vi "pace measurement_mso7014b.vi"(8 "error in (no error)":errorcluster, 11 "VISA resource name":refnum<visa-resource-name>) -> (0 "CH3 Waveform":waveform(dbl)(graph), 1 "CH1 Waveform":waveform(dbl)(graph), 2 "添加的数组":waveform(dbl)[](array[waveform]))   [LabVIEW 2016]
uses:
  <instrlib>/Agilent 6000 Series/Public/Data/Read Waveform Measurement.vi
  <instrlib>/Agilent 6000 Series/Agilent 6000 Series.lvlib
panel:
  out "Pluse Frequency":dbl
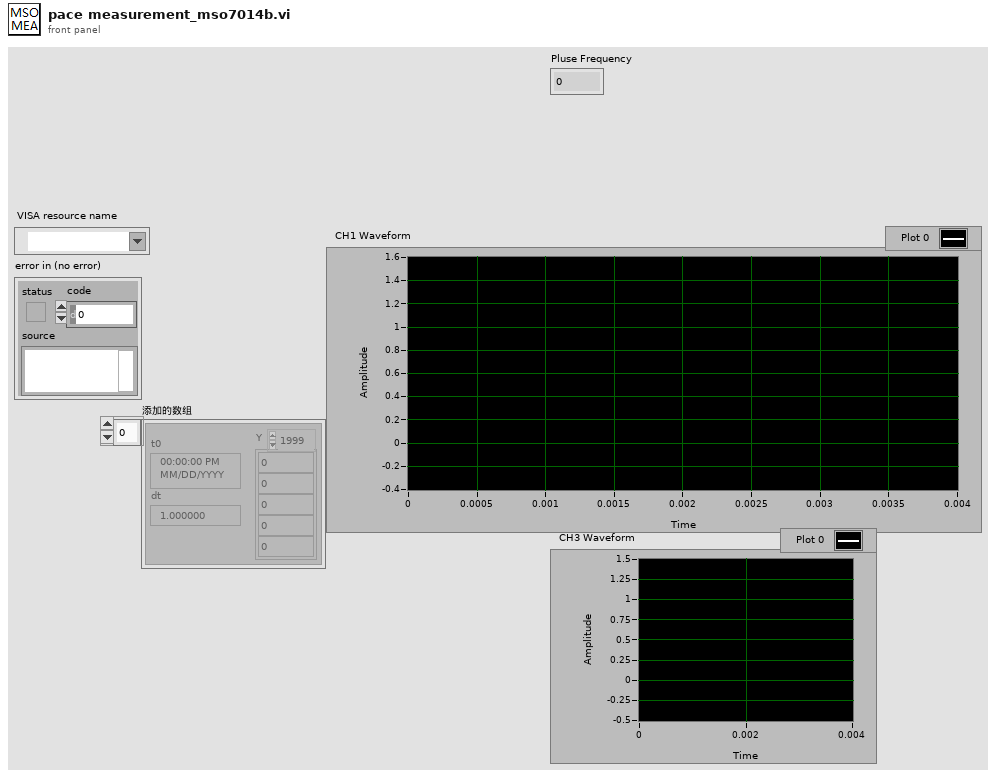
[diagram p1: front panel]
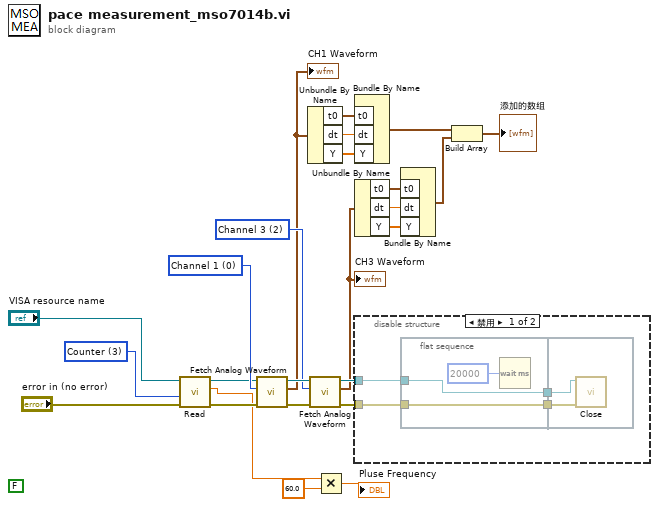
[diagram p0: block diagram]
diagram:
  w8 = u16 3 items=["Amplitude", "Voltage Average", "Base", "Counter", "Delay", "Duty Cycle", "Fall Time", "Frequency", "Voltage Max", "Voltage Min", "Overshoot", "Voltage Vpp", "Period", "Phase", "Preshoot", "Rise Time", "Voltage RMS", "Top", "Width Positive", "X at Max Y", "X at Min Y"] ("Measurement Function (7: Frequency)")
  (unwired) FALSE ("Continuous Acquisition Mode (T: Enable)")
  w23 = u16 2 items=["Channel 1", "Channel 2", "Channel 3", "Channel 4", "Math"] ("Source (0: Channel 1)")
  w25 = u16 0 items=["Channel 1", "Channel 2", "Channel 3", "Channel 4", "Math"] ("Source (0: Channel 1)")
  n1 = call-poly <instrlib>:"Read.vi"("error in (no error)"="error in (no error)", "Measurement Function (7: Frequency)"=w8, "VISA resource name"="VISA resource name") -> ("error out"=w4:errorcluster, "Measured Value"=w3:dbl, "VISA resource name out"=w6:refnum<visa-resource-name>)  [unwired: 6 in]
  n2 = call <instrlib>:"Fetch Analog Waveform.vi"("error in (no error)"=w4, "Source (0: Channel 1)"=w25, "VISA resource name"=w6) -> ("error out"=w20:errorcluster, "Waveform Data"=w19:waveform(dbl), "VISA resource name out"=w24:refnum<visa-resource-name>)  [unwired: 6 in]
  "CH1 Waveform" <- w19
  n3 = Unbundle By Name(w19) -> ("t0"=w18:timestamp, "dt"=w17:dbl, "Y"=w16:dbl[])
  n4 = call <instrlib>:"Fetch Analog Waveform.vi"("error in (no error)"=w20, "Source (0: Channel 1)"=w23, "VISA resource name"=w24) -> ("error out"=w21:errorcluster, "Waveform Data"=w12:waveform(dbl), "VISA resource name out"=w22:refnum<visa-resource-name>)  [unwired: 6 in]
  "CH3 Waveform" <- w12
  n5 = Multiply(x=w3, y=60.0) -> (x*y=→"Pluse Frequency":dbl)
  n6 = Bundle By Name("t0"=w18, "dt"=w17, "Y"=w16) -> (w11:waveform(dbl))  [unwired: 1 in]
  n7 = Unbundle By Name(w12) -> ("t0"=w13:timestamp, "dt"=w14:dbl, "Y"=w15:dbl[])
  n8 = disable-structure shown="禁用" {
    disable-tunnel: w22 -> [w27 _]
    disable-tunnel: w21 -> [w26 _]
    frame Disabled {
      n9 = flat-sequence {
        tunnel: w26 -> [w31]
        tunnel: w27 -> [w32]
        tunnel: [w32] -> w29
        tunnel: [w31] -> w28
        tunnel: w29 -> [w34]
        tunnel: w28 -> [w33]
        frame #0 {
          n10 = Wait (ms)(milliseconds to wait=u32 20000 ("等待时间（毫秒）")) -> ()  [unwired: 1 out]
        }
        frame #1 {
          n11 = call <instrlib>:"Close.vi"("error in (no error)"=w33, "VISA resource name"=w34) -> ()  [unwired: 9 in, 1 out]
        }
      }
    }
    frame Enabled {
    }
  }
  n12 = Bundle By Name("t0"=w13, "dt"=w14, "Y"=w15) -> (w10:waveform(dbl))  [unwired: 1 in]
  n13 = Build Array(w11, w10) -> (→"添加的数组":waveform(dbl)[])
